vi "Sample Transfer Set Heater.vi"(7 "Container":T1, 8 "error in (no error)":errorcluster, 10 "ON/OFF(OFF)":bool, 11 "cRIO-CO2 in":refnum<class "cRIO-CO2.lvclass">) -> (0 "error out":errorcluster, 2 "Container Name String":string, 3 "cRIO-CO2 out":refnum<class "cRIO-CO2.lvclass">)   [LabVIEW 2015, in "cRIO-Carbondioxide.lvlib" / "cRIO-CO2.lvlib" / "cRIO-CO2.lvclass"]
uses:
  cRIO-CO2.lvclass
  Controls/Sample Transfer Container Enumerator.ctl
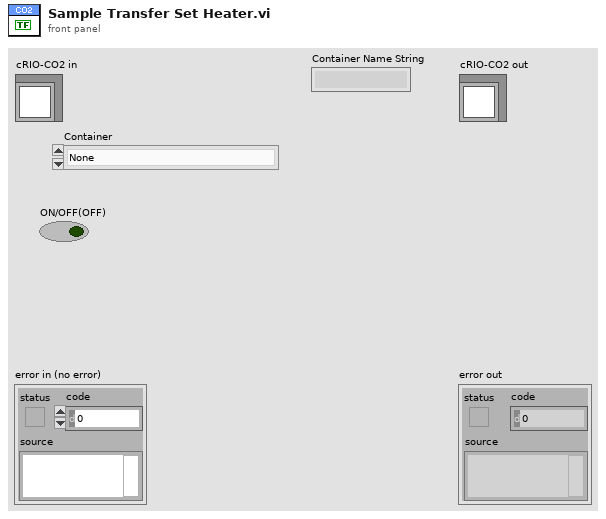
[diagram p1: front panel]
types:
  T1 = typedef "Sample Transfer Container Enumerator.ctl" = enum16{"None", "Sample 1", "Sample 2", "Sample 3", "Sample 4", "Sample 5", "Storage 01", "Storage 02", "Storage 03", "Storage 04", "Storage 05", "Storage 06", "Storage 07", "Storage 08", "Storage 09", "Storage 10", "Storage 11", "Storage 12", "Syringe", "Undefined"}
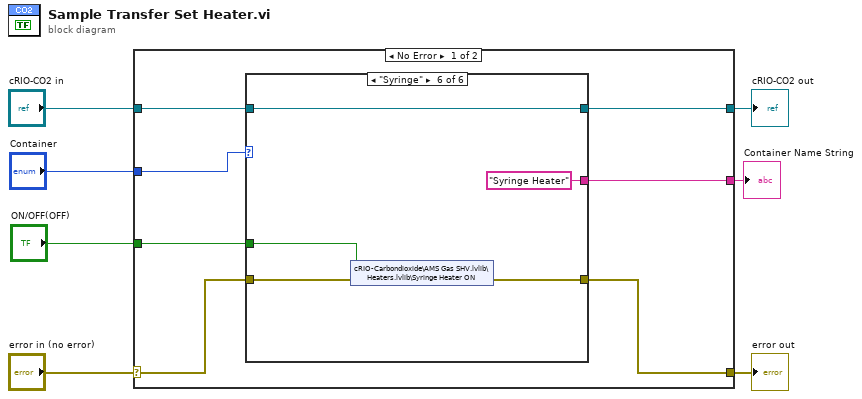
[diagram p0: block diagram]
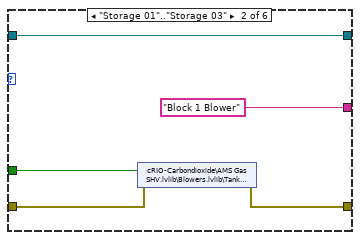
[diagram p3: hidden frame]
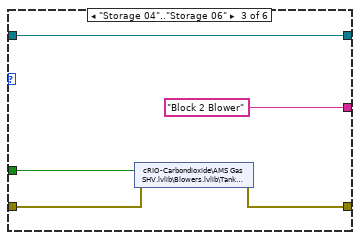
[diagram p4: hidden frame]
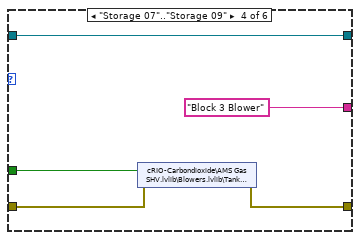
[diagram p5: hidden frame]
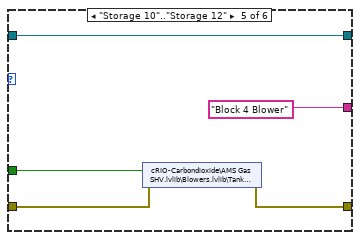
[diagram p6: hidden frame]
diagram:
  n1 = case shown="No Error" "error in (no error)" {
    selector: "error in (no error)" -> [w8 w43]
    tunnel: [w13 w43] -> w6
    tunnel: [w14 w42] -> w4
    tunnel: "cRIO-CO2 in" -> [w12 w42]
    tunnel: "Container" -> [w11 _]
    tunnel: "ON/OFF(OFF)" -> [w10 _]
    tunnel: [w9 _] -> w1
    frame No Error {
      n2 = case shown="\"Syringe\"" w11 {
        tunnel: w8 -> [w16 w19 w24 w29 w34 w39]
        tunnel: w12 -> [w15 w21 w26 w31 w36 w41]
        tunnel: [w16 w18 w23 w28 w33 w38] -> w13
        tunnel: [w15 w21 w26 w31 w36 w41] -> w14
        tunnel: w10 -> [_ w17 w22 w27 w32 w37]
        tunnel: [_ "Block 1 Blower" ("string") "Block 2 Blower" ("string") "Block 3 Blower" ("string") "Block 4 Blower" ("string") "Syringe Heater" ("string")] -> w9
        frame "None", Default {
        }
        frame "Storage 01".."Storage 03" {
          n3 = shared-variable "cRIO-Carbondioxide\\AMS Gas SHV.lvlib\\Blowers.lvlib\\Tank Blower 1"(w17, error in=w19) -> (error out=w18:errorcluster)
        }
        frame "Storage 04".."Storage 06" {
          n4 = shared-variable "cRIO-Carbondioxide\\AMS Gas SHV.lvlib\\Blowers.lvlib\\Tank Blower 2"(w22, error in=w24) -> (error out=w23:errorcluster)
        }
        frame "Storage 07".."Storage 09" {
          n5 = shared-variable "cRIO-Carbondioxide\\AMS Gas SHV.lvlib\\Blowers.lvlib\\Tank Blower 3"(w27, error in=w29) -> (error out=w28:errorcluster)
        }
        frame "Storage 10".."Storage 12" {
          n6 = shared-variable "cRIO-Carbondioxide\\AMS Gas SHV.lvlib\\Blowers.lvlib\\Tank Blower 4"(w32, error in=w34) -> (error out=w33:errorcluster)
        }
        frame "Syringe" {
          n7 = shared-variable "cRIO-Carbondioxide\\AMS Gas SHV.lvlib\\Heaters.lvlib\\Syringe Heater ON"(w37, error in=w39) -> (error out=w38:errorcluster)
        }
      }
    }
    frame Error {
    }
  }
  "error out" <- w6
  "cRIO-CO2 out" <- w4
  "Container Name String" <- w1
